vi "Update App Version.vi"(8 "error in (no error)":errorcluster, 10 "App Version String":string, 11 "Builder in":refnum<class "Builder.lvclass">) -> (0 "error out":errorcluster, 3 "Builder out":refnum<class "Builder.lvclass">)   [LabVIEW 2020, in "Builder Tools.lvlib" / "Builder.lvclass"]
uses:
  Builder.lvclass
  Builder.lvclass/Builder.ctl
  Builder Core/App Version.vi
  Builder Core/Builder Core.lvlib
  <vilib>/Utility/traverseref.llb/TRef TravTarget.ctl
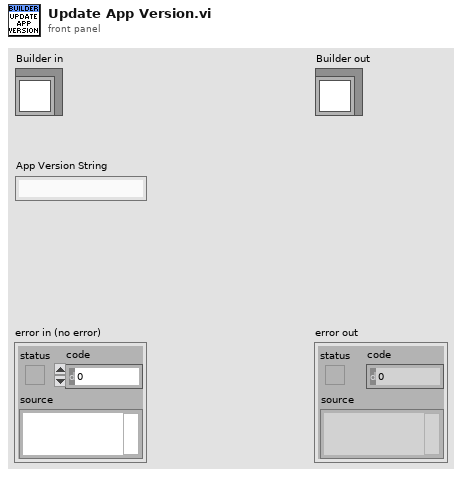
[diagram p1: front panel]
types:
  T1 = typedef "TRef TravTarget.ctl" = enum16{"FP", "BD", "Other"}
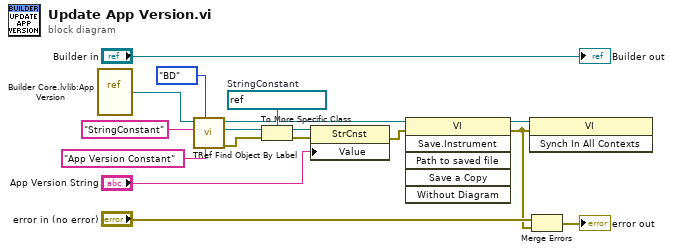
[diagram p0: block diagram]
diagram:
  w9 = refnum<vi> refnum  # StringConstant
  n1 = vi-ref "Builder Core.lvlib:App Version.vi"() -> (w15:refnum<vi>)
  n2 = call <vilib>:"TRef Find Object By Label.vi"("Label"="App Version Constant", "Traverse Target"=TRef_TravTarget."BD", "Class Name"="StringConstant", "VI Ref"=w15) -> ("error out"=w10:errorcluster, "Found Obj Ref"=w11:refnum<vi>, "dup VI Ref"=w5:refnum<vi>)  [unwired: 4 in, 1 out]
  n3 = To More Specific Class(target class=w9, reference=w11, error in=w10) -> (specific class reference=w8:refnum<vi>, error out=w7:errorcluster)
  n4 = property class="StrCnst"(reference=w8, error in=w7, "Value"="App Version String") -> (error out=w4:errorcluster)  [unwired: 1 out]
  n5 = invoke class="VI" method="Save.Instrument"(reference=w5, error in=w4) -> (reference out=w3:refnum<vi>, error out=w1:errorcluster)  [unwired: 4 in, 4 out]
  n6 = invoke class="VI" method="Synch In All Contexts"(reference=w3, error in=w1) -> ()  [unwired: 1 in, 3 out]
  n7 = Merge Errors("error in (no error)", w1) -> (→"error out":errorcluster)
  "Builder out" <- "Builder in"
